vi "setEventId.vi"(8 "error in (no error)":errorcluster, 10 "eventId":dbl, 11 "RfRamp in":refnum<class "RfRamp.lvclass">) -> (0 "error out":errorcluster, 3 "RfRamp out":refnum<class "RfRamp.lvclass">)   [LabVIEW 2009, in "Tools.lvlib" / "Scripting.lvlib" / "RfRamp.lvclass"]
uses:
  RfRamp.lvclass
  Rf Event/rf.lvclass
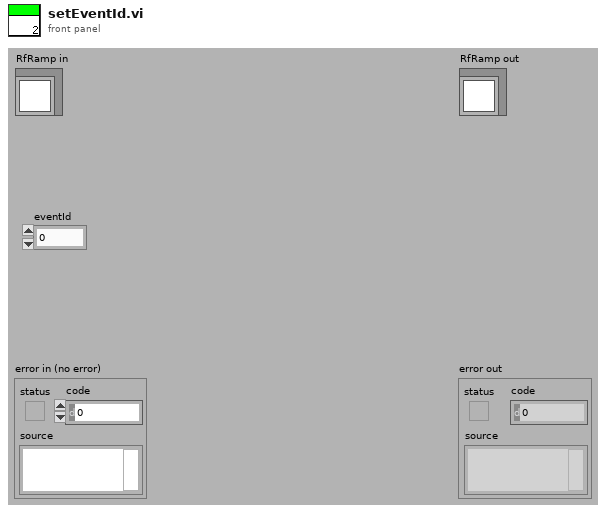
[diagram p1: front panel]
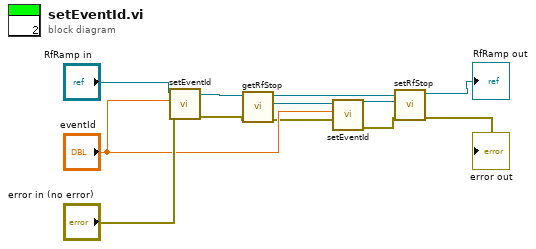
[diagram p0: block diagram]
diagram:
  n1 = call-parent "setEventId.vi"("error in (no error)"="error in (no error)", "eventId"="eventId", "ScriptEvent in"="RfRamp in") -> ("error out"=w8:errorcluster, "ScriptEvent out"=w9:refnum<class "RfRamp.lvclass">)  [unwired: 7 in]
  n2 = call "getRfStop.vi"("error in (no error)"=w8, "RfRamp in"=w9) -> ("error out"=w4:errorcluster, "rfStop"=w5:refnum<class "rf.lvclass">, "RfRamp out"=w7:refnum<class "RfRamp.lvclass">)  [unwired: 7 in]
  n3 = call-parent "setEventId.vi"("error in (no error)"=w4, "eventId"="eventId", "ScriptEvent in"=w5) -> ("error out"=w3:errorcluster, "ScriptEvent out"=w6:refnum<class "rf.lvclass">)  [unwired: 7 in]
  n4 = call "setRfStop.vi"("error in (no error)"=w3, "rfStop"=w6, "RfRamp in"=w7) -> ("error out"=→"error out":errorcluster, "RfRamp out"=→"RfRamp out":refnum<class "RfRamp.lvclass">)  [unwired: 7 in]
